vi "MeasToTable (SubVI).vi"(6 "UNDT_NTick":i32, 9 "Meas":T1 {"FFT amplitude mean" format="%.2p"; "DC" format="%0.2p"; "time trig 2" format="%0.2p"; "time trig" format="%0.2p"; "detected frequency 2" format="%.2p"; "way sensor 2" format="%.2p"; "way sensor 1" format="%.2p"; "detected frequency" format="%.2p"; "RMS" format="%0.2p"; "amplitude" format="%.2p"; "FFT amplitude" format="%.2p"}, 10 "N tick":u8, 11 "Table":string[][](array[string])=[["Частота, МГц", "1", "4998611", "4999874"], ["СКЗ, В", "1", "1.426E-5", "1.120E-1"], ["Амплитуда, В", "1", "2.016E-5", "1.583E-1"], ["Амплитуда, дБмкВ", "1", "26.09", "103.99"], ["Датчик пути 1, мм", "1", "0.0", "-0.2"], ["Датчик пути 2, мм", "1", "-0.3", "-0.3"], ["Время, сек", "1", "8.000E-5", "8.000E-5"]]) -> (3 "TableOut":string[][](array[string]))   [LabVIEW 2017]
uses:
  Control_EU/MeasControl.ctl
  Global_SNK3_HF.vi
panel:
  out "x-y*floor(x/y)":u8
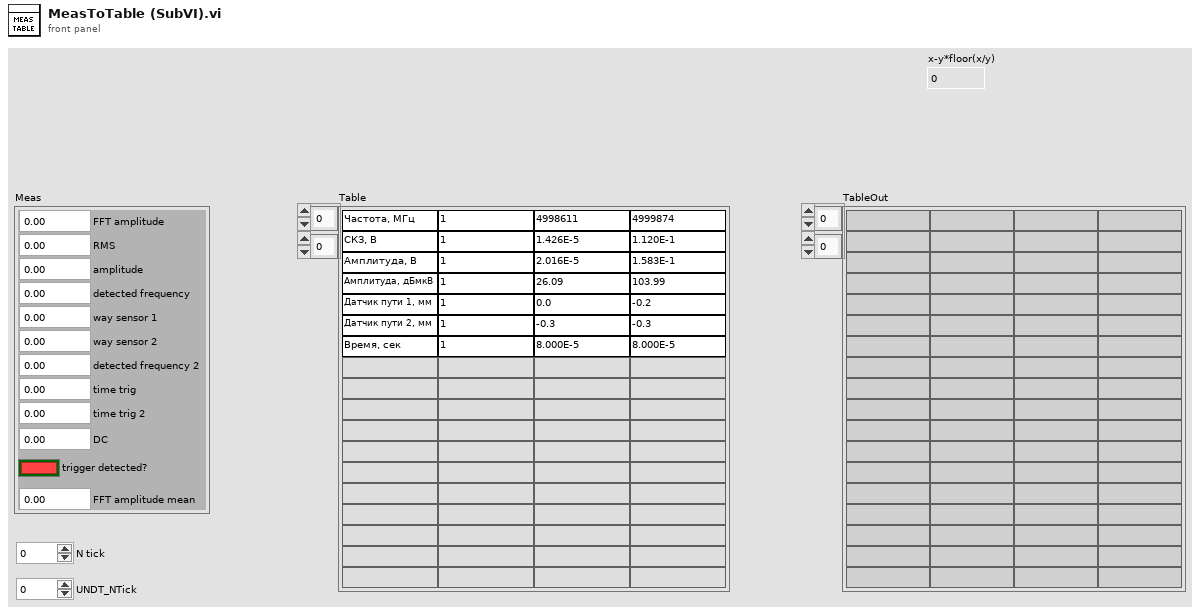
[diagram p1: front panel]
types:
  T1 = typedef "MeasControl.ctl" = cluster{"FFT amplitude":dbl, "amplitude":dbl, "RMS":dbl, "detected frequency":dbl, "way sensor 1":ext, "way sensor 2":ext, "detected frequency 2":dbl, "time trig":dbl, "time trig 2":dbl, "DC":dbl, "trigger detected?":bool, "FFT amplitude mean":dbl}
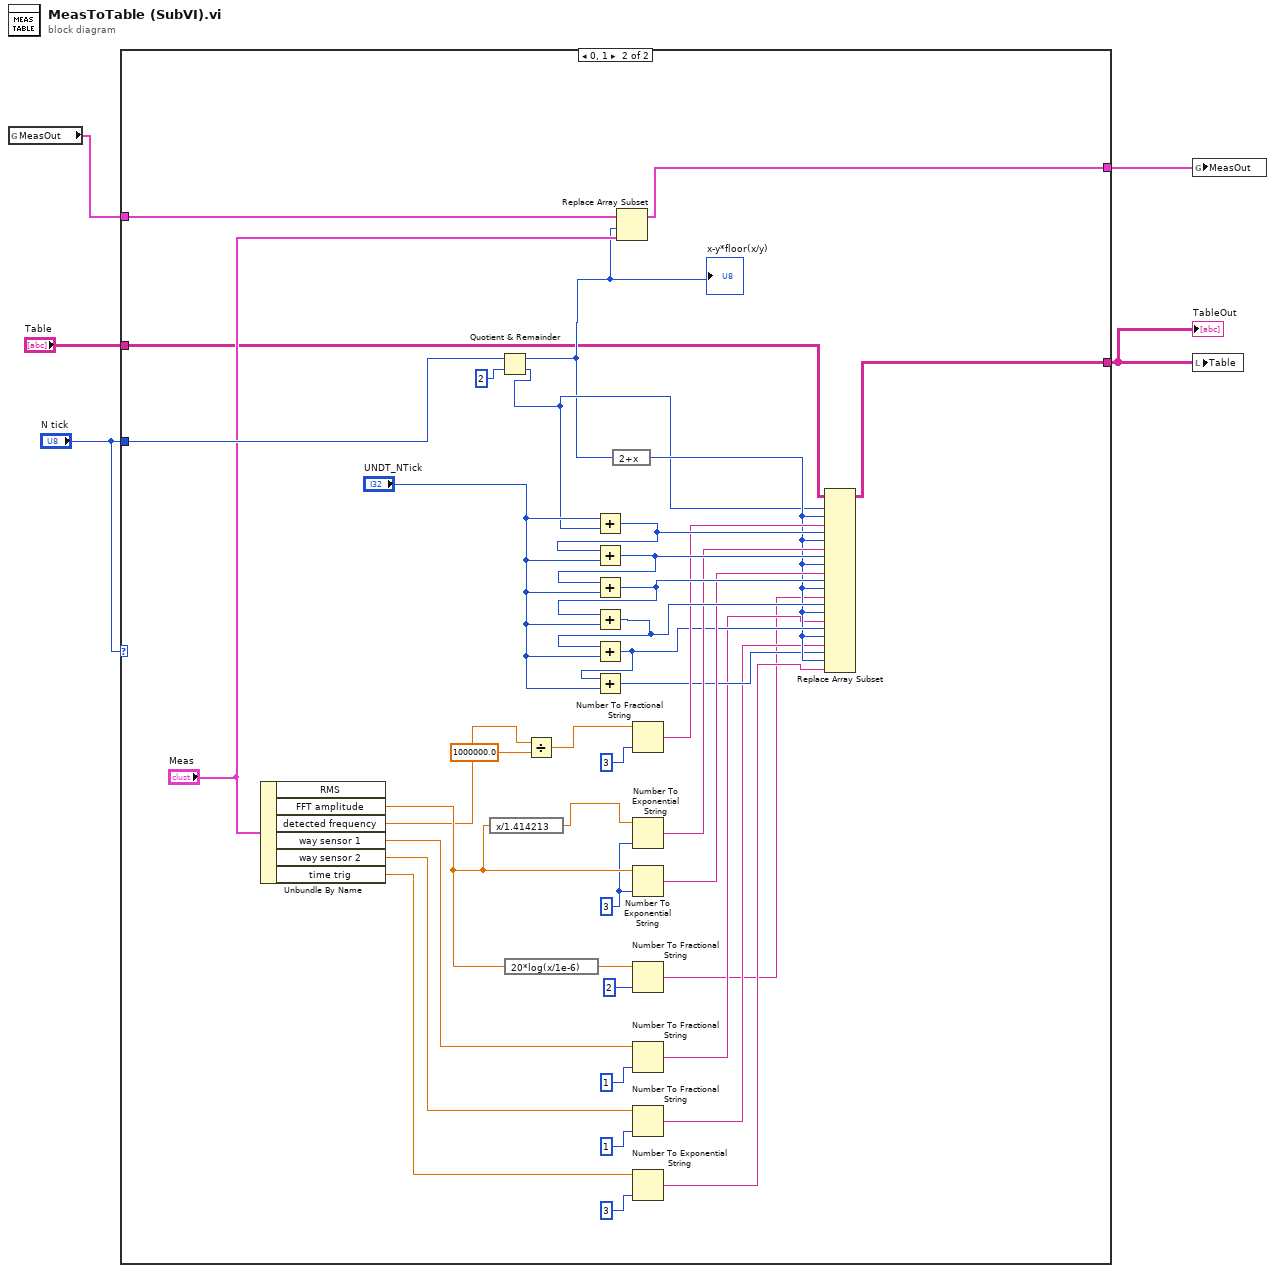
[diagram p0: block diagram]
diagram:
  n1 = global read "Global_SNK3_HF.vi" "MeasOut"() -> (w4:T1[])
  n2 = case shown="0, 1" "N tick" {
    tunnel: "N tick" -> [_ w45]
    tunnel: w4 -> [w7 w11]
    tunnel: [w7 w10] -> w3
    tunnel: [w6 w9] -> w2
    tunnel: "Table" -> [w6 w8]
    frame 2, Default {
    }
    frame 0, 1 {
      w18 = i16 3 ("precision (6)")
      n3 = Unbundle By Name("Meas") -> ("FFT amplitude"=w20:dbl, "detected frequency"=w14:dbl, "way sensor 1"=w39:ext, "way sensor 2"=w38:ext, "time trig"=w36:dbl)  [unwired: 1 out]
      n4 = expression code="x/1.414213"(w20) -> (w19:dbl)
      n5 = Quotient & Remainder(x=w45, y=u8 2) -> (x-y*floor(x/y)=w15:u8, floor(x/y)=w17:u8)
      "x-y*floor(x/y)" <- w15
      n6 = expression code="20*log(x/1e-6)"(w20) -> (w30:dbl)
      n7 = Divide(x=w14, y=1000000.0) -> (x/y=w12:dbl)
      n8 = Add(x="UNDT_NTick", y=w17) -> (x+y=w43:i32)
      n9 = Add(x=w43, y="UNDT_NTick") -> (x+y=w42:i32)
      n10 = Add(x=w42, y="UNDT_NTick") -> (x+y=w35:i32)
      n11 = Add(x=w35, y="UNDT_NTick") -> (x+y=w34:i32)
      n12 = Add(x=w34, y="UNDT_NTick") -> (x+y=w28:i32)
      n13 = Add(x=w28, y="UNDT_NTick") -> (x+y=w25:i32)
      n14 = expression code="2+x"(w15) -> (w26:u8)
      n15 = Replace Array Subset(array=w11, new element="Meas", index=w15) -> (w10:T1[])
      n16 = Number To Fractional String(number=w12, precision (6)=i16 3) -> (F-format string=w33:string)  [unwired: 2 in]
      n17 = Number To Exponential String(number=w19, precision (6)=w18) -> (E-format string=w31:string)  [unwired: 2 in]
      n18 = Number To Exponential String(number=w20, precision (6)=w18) -> (E-format string=w32:string)  [unwired: 2 in]
      n19 = Number To Fractional String(number=w30, precision (6)=i16 2) -> (F-format string=w21:string)  [unwired: 2 in]
      n20 = Number To Fractional String(number=w39, precision (6)=i16 1) -> (F-format string=w22:string)  [unwired: 2 in]
      n21 = Number To Fractional String(number=w38, precision (6)=i16 1) -> (F-format string=w23:string)  [unwired: 2 in]
      n22 = Number To Exponential String(number=w36, precision (6)=i16 3) -> (E-format string=w24:string)  [unwired: 2 in]
      n23 = Replace Array Subset(array=w8, new element #1=w33, index (row) #1=w17, index (col) #1=w26, new element #2=w31, index (row) #2=w43, index (col) #2=w26, new element #3=w32, index (row) #3=w42, index (col) #3=w26, new element #4=w21, index (row) #4=w35, index (col) #4=w26, new element #5=w22, index (row) #5=w34, index (col) #5=w26, new element #6=w23, index (row) #6=w28, index (col) #6=w26, new element #7=w24, index (row) #7=w25, index (col) #7=w26) -> (w9:string[][])
    }
  }
  "TableOut" <- w2
  n24 = global write "Global_SNK3_HF.vi" "MeasOut"(w3) -> ()
  n25 = local write "Table"(w2) -> ()
